vi "chconfigset.vi"(7 "Enum":enum16{"init", "read", "treeheader", "ctrrefin"}(ring)=enum."read", 9 "ref":refnum<vi>[](array[refnum]), 10 "chtree config":T1={"ch"=[{"String"="通道名", "use"=TRUE, "display"=0, "Enum"=enum."Chname"}, {"String"="使用", "use"=TRUE, "display"=0, "Enum"=enum."USE"}, {"String"="频率", "use"=TRUE, "display"=0, "Enum"=enum."fre"}, {"String"="增益", "use"=TRUE, "display"=0, "Enum"=enum."range"}, {"String"="传感器型号", "use"=TRUE, "display"=0, "Enum"=enum."senNO"}, {"String"="物理量", "use"=TRUE, "display"=0, "Enum"=enum."PHname"}, {"String"="单位", "use"=TRUE, "display"=0, "Enum"=enum."unit"}, {"String"="校准类别", "use"=TRUE, "display"=0, "Enum"=enum."CALclass"}, {"String"="校准系数", "use"=TRUE, "display"=0, "Enum"=enum."K"}, {"String"="样准偏移量", "use"=TRUE, "display"=0, "Enum"=enum."OFF"}, {"String"="报警", "use"=TRUE, "display"=0, "Enum"=enum."Alrm"}, {"String"="滤波", "use"=TRUE, "display"=0, "Enum"=enum."filt"}, {"String"="电源供电", "use"=TRUE, "display"=0, "Enum"=enum."Power"}, {"String"="显示", "use"=TRUE, "display"=0, "Enum"=enum."display"}, {"String"="报警判断", "use"=TRUE, "display"=0, "Enum"=enum."compare"}, {"String"="判断值", "use"=TRUE, "display"=0, "Enum"=enum."threshold"}, {"String"="信号类型", "use"=TRUE, "display"=0, "Enum"=enum."Etype"}], "displya num"=1, "range value"=["0~10V", "0~5V", "±10V", "±5V", "", "", "", "", "", "", "", "", "", "", "", "", "", "", "", ""], "Etype"=["0~10V", "0~5V", "±10V", "±5V", "", "", "", "", "", "", "", "", "", "", "", "", "", "", "", ""], "CLASS"=[enum."CNO", enum."CName", enum."ClassI"]}) -> (0 "All ref":refnum<vi>[](array[refnum]), 1 "ref out":refnum<vi>[](array[refnum]), 2 "chtree config out":T1, 3 "tree header":string[](array[string]))   [LabVIEW 2011]
uses:
  chtype.ctl
  config table enum.ctl
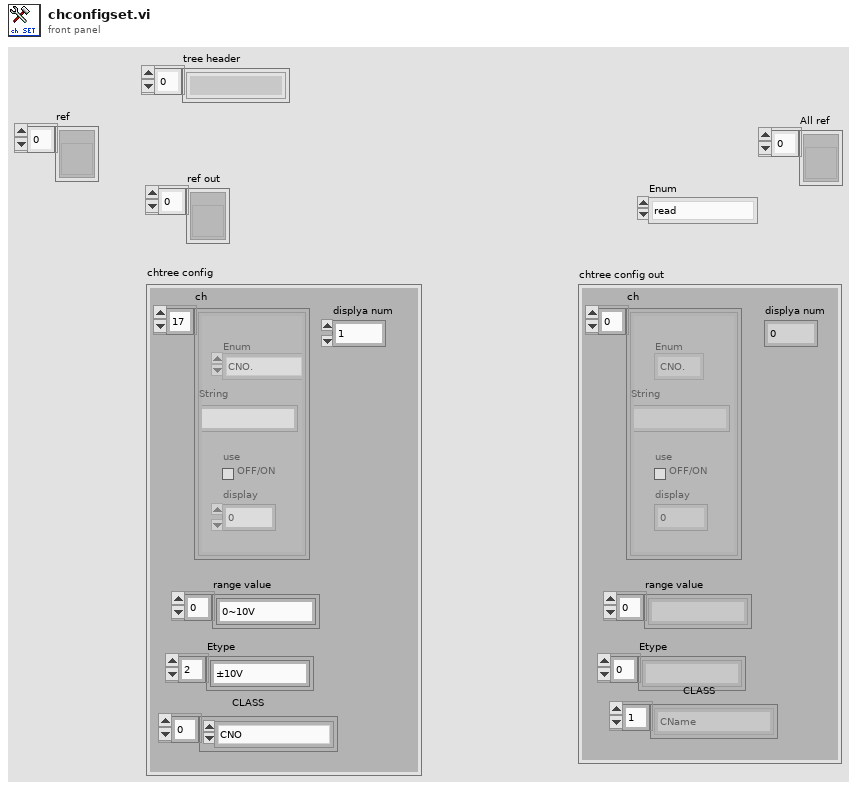
[diagram p1: front panel]
types:
  T1 = typedef "chtype.ctl" = cluster{"ch":cluster{"String":string, "use":bool, "display":u16, "Enum":T2}[], "displya num":i32, "range value":string[], "Etype":string[], "CLASS":enum16{"CName", "CNO", "ClassI", "ClassII"}[]}
  T2 = typedef "config table enum.ctl" = enum16{"CNO.", "CName", "CLASSI", "CLASSII", "ch", "Chname", "USE", "fre", "range", "senNO", "PHname", "unit", "CALclass", "K", "OFF", "Alrm", "filt", "Power", "display", "threshold", "compare", "Etype"}
  T3 = cluster{"String":string, "use":bool, "display":u16, "Enum":T2}[]
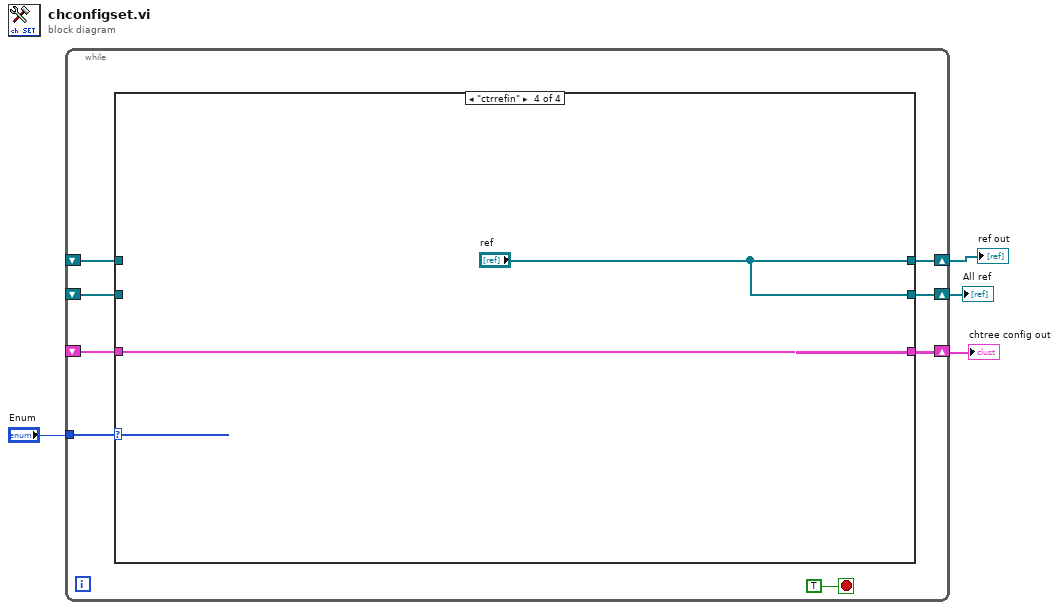
[diagram p0: block diagram]
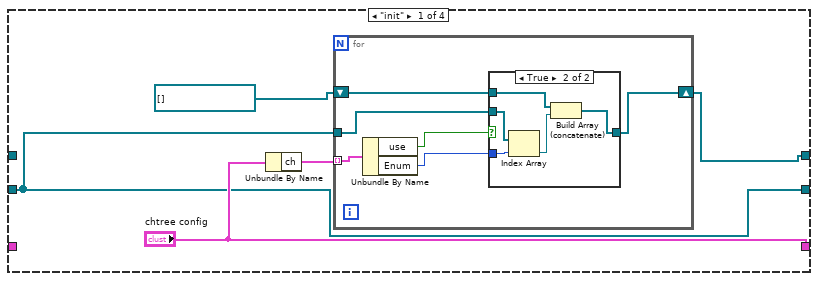
[diagram p2: hidden frame]
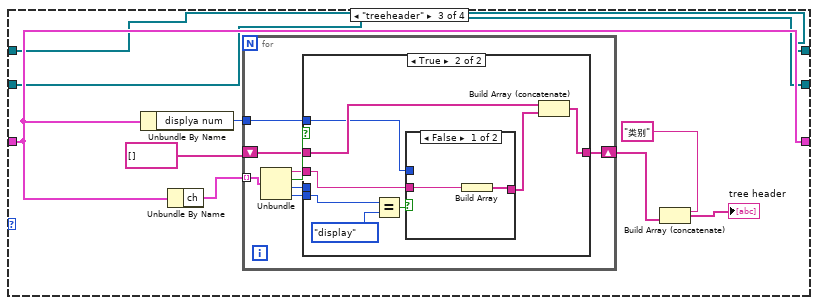
[diagram p5: hidden frame]
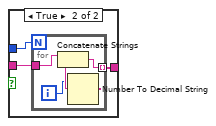
[diagram p7: hidden frame]
diagram:
  n1 = while {
    shift-right: [w12] -> w3
    shift-left: _ -> [w9]
    tunnel: "Enum" -> [w10]
    shift-right: [w8] -> w2
    shift-left: _ -> [w7]
    shift-right: [w6] -> w1
    shift-left: _ -> [w5]
    stop <- TRUE stop-if-true
    n2 = case shown="\"ctrrefin\"" w10 {
      tunnel: ["chtree config" w32 w35 w69] -> w12
      tunnel: w9 -> [_ w32 w35 w69]
      tunnel: [w14 w31 w34 "ref"] -> w8
      tunnel: w7 -> [_ w31 w34 _]
      tunnel: [w13 w30 w33 "ref"] -> w6
      tunnel: w5 -> [w13 w30 w33 _]
      frame "init" {
        n3 = Unbundle By Name("chtree config") -> ("ch"=w16:T3)
        n4 = for {
          tunnel: w16 -> [w23] mode=indexing
          tunnel: w13 -> [w21]
          shift-right: [w20] -> w14
          shift-left: refnum<vi>[] [] ("ref") -> [w18]
          n5 = Unbundle By Name(w23) -> ("use"=w22:bool, "Enum"=w19:T2)
          n6 = case shown="True" w22 {
            tunnel: w21 -> [_ w29]
            tunnel: [w24 w25] -> w20
            tunnel: w19 -> [_ w28]
            tunnel: w18 -> [w24 w27]
            frame False {
            }
            frame True {
              n7 = Index Array(array=w29, index=w28) -> (element=w26:refnum<vi>)
              n8 = Build Array (concatenate)(w27, w26) -> (w25:refnum<vi>[])
            }
          }
        }
      }
      frame "read", Default {
      }
      frame "treeheader" {
        n9 = Unbundle By Name(w35) -> ("displya num"=w37:i32)
        n10 = Unbundle By Name(w35) -> ("ch"=w41:T3)
        n11 = for {
          tunnel: w41 -> [w49] mode=indexing
          shift-right: [w46] -> w40
          shift-left: string[] [] -> [w47]
          tunnel: w37 -> [w42]
          n12 = Unbundle(w49) -> ("String"=w45:string, "use"=w48:bool, "display"=w43:u16, "Enum"=w44:T2)
          n13 = case shown="True" w48 {
            tunnel: w47 -> [w50 w58]
            tunnel: [w50 w57] -> w46
            tunnel: w45 -> [_ w53]
            tunnel: w44 -> [_ w56]
            tunnel: w43 -> [_ _]
            tunnel: w42 -> [_ w51]
            frame False {
            }
            frame True {
              n14 = Equal?(x=w56, y=config_table_enum."display") -> (x = y?=w54:bool)
              n15 = case shown="False" w54 {
                tunnel: w53 -> [w60 w61]
                tunnel: [w59 w62] -> w52
                tunnel: w51 -> [_ w63]
                frame False {
                  n16 = Build Array(w60) -> (w59:string[])
                }
                frame True {
                  n17 = for {
                    N: w63 -> [_]
                    tunnel: [w67] -> w62 mode=indexing
                    tunnel: w61 -> [w66]
                    i -> [w64]
                    n18 = Number To Decimal String(number=w64) -> (decimal integer string=w65:string)  [unwired: 1 in]
                    n19 = Concatenate Strings(w66, w65) -> (w67:string)
                  }
                }
              }
              n20 = Build Array (concatenate)(w58, w52) -> (w57:string[])
            }
          }
        }
        n21 = Build Array (concatenate)("类别", w40) -> (→"tree header":string[])
      }
      frame "ctrrefin" {
      }
    }
  }
  "chtree config out" <- w3
  "ref out" <- w2
  "All ref" <- w1
